vi "Get PSQL datatype.vi"(8 "error in (no error)":errorcluster, 9 "Column":string, 10 "Table":string, 11 "LV-Data.PGSQL in":refnum<class "LV-Data.PGSQL.lvclass">) -> (0 "error out":errorcluster, 2 "Get:Get String":string, 3 "LV-Data.PGSQL out":refnum<class "LV-Data.PGSQL.lvclass">)   [LabVIEW 2016]
uses:
  LV-Data/src/LV-Data.PG/LV-Data.PGSQL.lvclass
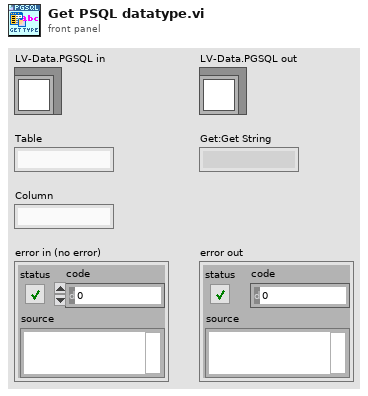
[diagram p1: front panel]
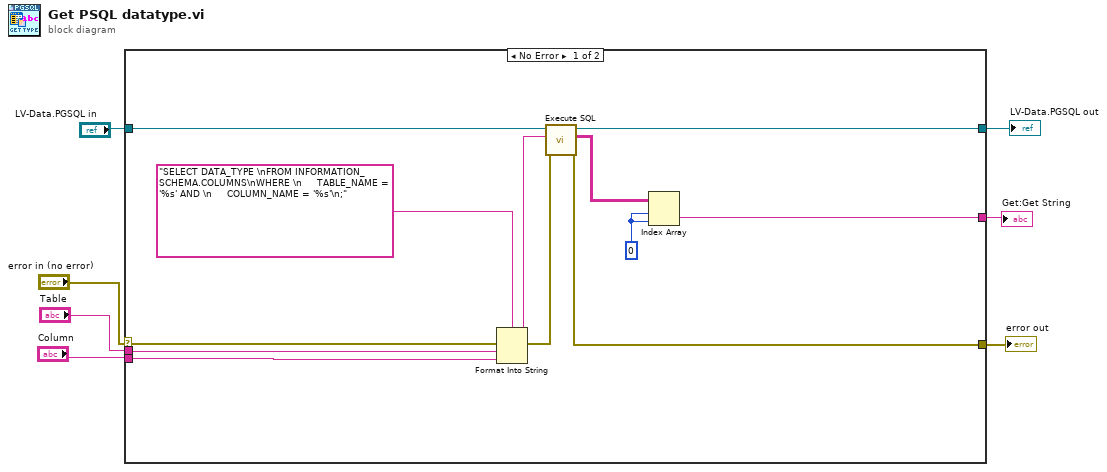
[diagram p0: block diagram]
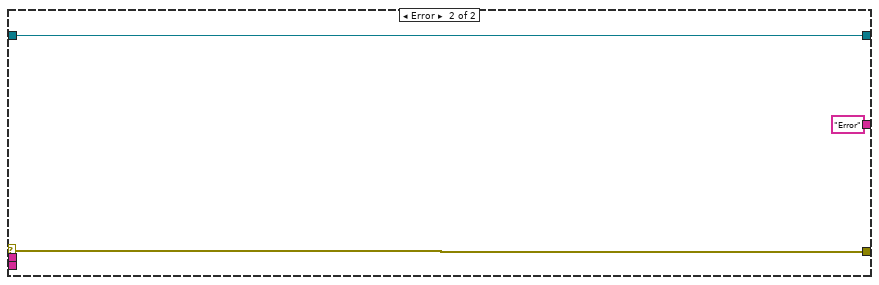
[diagram p2: hidden frame]
diagram:
  n1 = case shown="No Error" "error in (no error)" {
    selector: "error in (no error)" -> [w11 w21]
    tunnel: "Column" -> [w13 _]
    tunnel: "LV-Data.PGSQL in" -> [w12 w22]
    tunnel: [w9 w21] -> w7
    tunnel: [w10 w22] -> w4
    tunnel: "Table" -> [w14 _]
    tunnel: [w8 "Error" ("Get:Get String")] -> w5
    frame No Error {
      w17 = 0 ("index (row)")
      n2 = Format Into String(format string="SELECT DATA_TYPE \nFROM INFORMATION_SCHEMA.COLUMNS\nWHERE \n     TABLE_NAME = '%s' AND \n     COLUMN_NAME = '%s'\n;", error in=w11, w14, w13) -> (resulting string=w15:string, error out=w16:errorcluster)  [unwired: 1 in]
      n3 = call "Execute SQL.vi"("error in"=w16, "SQL"=w15, "Data.PG"=w12) -> ("error out"=w9:errorcluster, "Result"=w19:string[][], "Data.PG out"=w10:refnum<class "LV-Data.PGSQL.lvclass">)  [unwired: 6 in]
      n4 = Index Array(array=w19, index (row)=w17, index (col)=w17) -> (element=w8:string)
    }
    frame Error {
    }
  }
  "error out" <- w7
  "Get:Get String" <- w5
  "LV-Data.PGSQL out" <- w4
